vi "Ring Counter 8 Bit (SubVI).vi"(7 "Increment":u8=1) -> (0 "Next Count":u8, 1 "Count":u8, 3 "End of Count?":bool)   [LabVIEW 2014]
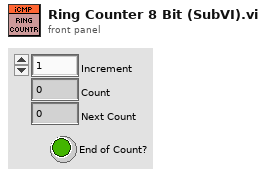
[diagram p1: front panel]
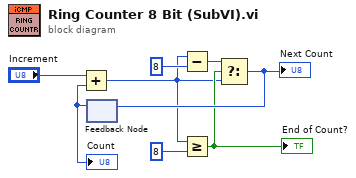
[diagram p0: block diagram]
diagram:
  n1 = feedback #1() -> (w3:u8)  [unwired: 1 in]
  "Count" <- w3
  n2 = Add(x="Increment", y=w3) -> (x+y=w4:u8)
  n3 = Subtract(x=w4, y=u8 8 ("x")) -> (x-y=w6:u8)
  n4 = Greater Or Equal?(x=w4, y=u8 8) -> (x >= y?=w7:bool)
  "End of Count?" <- w7
  n5 = Select(t=w6, s=w7, f=w4) -> (s? t:f=w8:u8)
  "Next Count" <- w8
  n6 = feedback-in #1(w8) -> ()
